vi "Msg.vi"(7 "Actor in":refnum<class "Actor.lvclass">, 11 "String Indicator Event in":refnum<class "String Indicator Msg.lvclass">) -> (5 "Actor out":refnum<class "Actor.lvclass">)   [LabVIEW 2021, in "String Indicator.lvlib" / "String Indicator Msg.lvclass"]
uses:
  String Indicator Msg.lvclass
  String Indicator/String Indicator.lvclass
  Actor/Actor/Actor.lvclass
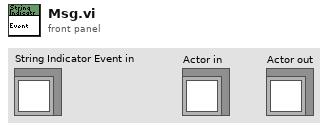
[diagram p1: front panel]
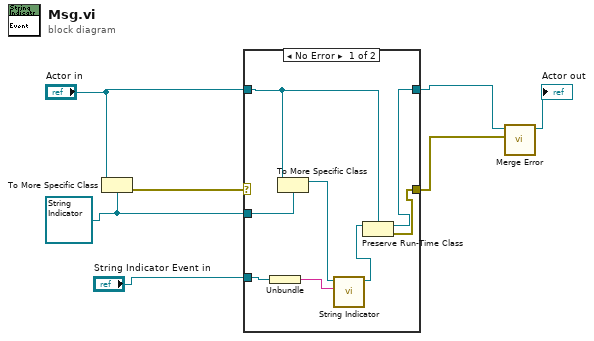
[diagram p0: block diagram]
diagram:
  w1 = refnum<class "String Indicator.lvclass"> refnum ("String Indicator Event.lvlib:String Indicator.lvclass")
  n1 = To More Specific Class(target class=w1, reference="Actor in") -> (error out=w7:errorcluster)  [unwired: 1 in, 1 out]
  n2 = case shown="No Error" w7 {
    selector: w7 -> [_ w16]
    tunnel: [w13 w17] -> w6
    tunnel: "Actor in" -> [w14 w17]
    tunnel: w1 -> [w15 _]
    tunnel: "String Indicator Event in" -> [w9 _]
    tunnel: [w12 w16] -> w5
    frame No Error {
      n3 = Unbundle(w9) -> (w8:string)
      n4 = To More Specific Class(target class=w15, reference=w14) -> (specific class reference=w11:refnum<class "String Indicator.lvclass">)  [unwired: 1 in, 1 out]
      n5 = call-dynamic "String Indicator.vi"("String Indicator"=w8, "String Indicator in"=w11) -> ("String Indicator out"=w10:refnum<class "String Indicator.lvclass">)  [unwired: 9 in]
      n6 = Preserve Run-Time Class(object in=w10, 2:w14) -> (object out=w13:refnum<class "Actor.lvclass">, error out=w12:errorcluster)  [unwired: 1 in]
    }
    frame Error {
    }
  }
  n7 = call-dynamic "Merge Error.vi"("Error"=w5, "Set Error in"=w6) -> ("Set Error out"=→"Actor out":refnum<class "Actor.lvclass">)  [unwired: 9 in]
